vi "Update Low Limit.vi"(7 "BLRL Type":T1, 8 "error in (no error)":errorcluster, 9 "Low Limit":string, 10 "Channel":string, 11 "BluelinesRedlines in":refnum<class "BluelinesRedlines.lvclass">) -> (0 "error out":errorcluster, 3 "BluelinesRedlines out":refnum<class "BluelinesRedlines.lvclass">)   [LabVIEW 2020, in "VolatusGUIElements.lvlib" / "BluelinesRedlines.lvclass"]
uses:
  BluelinesRedlines.lvclass
  BluelinesRedlines.lvclass/BluelinesRedlines.ctl
  User BluelinesRedlines/User BluelinesRedlines.lvclass
  C:/dev/lv20CE/relink/lv-volatus/VolatusGUI/BluelinesRedlines Source/BluelinesRedlines Source.lvclass
  VolatusGUI/BluelinesRedlines Source/BLRL Type.ctl
  VolatusGUI/BluelinesRedlines Source/BluelinesRedlines Source.lvclass
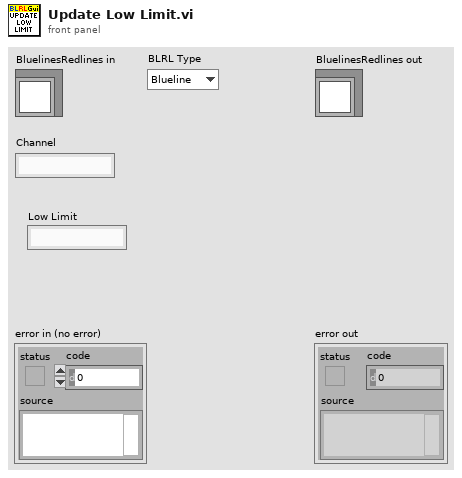
[diagram p1: front panel]
types:
  T1 = typedef "VolatusGUI.lvlib/BluelinesRedlines Source.lvclass/BLRL Type.ctl" = enum16{"Blueline", "Redline"}
  T2 = map{string, refnum<class "BluelinesRedlines Source.lvclass">}
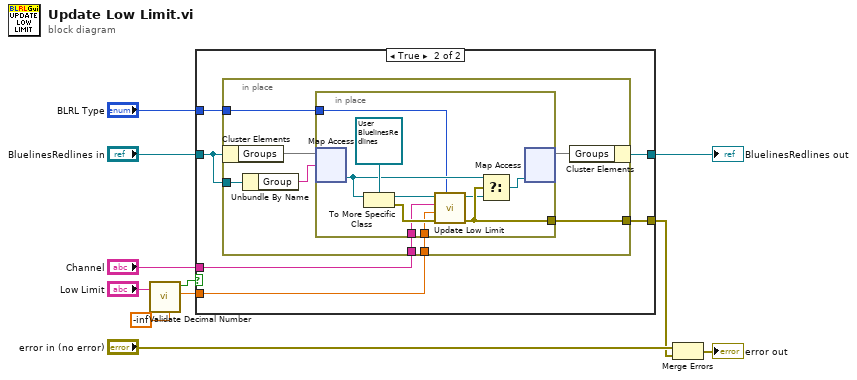
[diagram p0: block diagram]
diagram:
  n1 = call "Validate Decimal Number.vi"("String"="Low Limit", "Empty Default"=-inf) -> ("Valid"=w1:bool, "Value"=w3:dbl)  [unwired: 4 in]
  n2 = case shown="True" w1 {
    tunnel: "BluelinesRedlines in" -> [w12 w18]
    tunnel: [w12 w17] -> w9
    tunnel: "BLRL Type" -> [_ w16]
    tunnel: "Channel" -> [_ w15]
    tunnel: [_ w14] -> w4
    tunnel: w3 -> [_ w13]
    frame False {
    }
    frame True {
      n3 = in-place {
        in-place-border: w18 -> [w26]
        in-place-border: w15 -> [w22]
        in-place-border: w16 -> [w21]
        in-place-border: [w20] -> w14
        in-place-border: w13 -> [w19]
        n4 = in-place-cluster #1(w18) -> ("Groups"=w25:T2)
        n5 = Unbundle By Name(w26) -> ("Group"=w24:string)
        n6 = in-place {
          in-place-border: w22 -> [w30]
          in-place-border: w21 -> [w29]
          in-place-border: [w36] -> w20
          in-place-border: w19 -> [w27]
          n7 = in-place-map #2(w25, w24) -> (w33:refnum<class "BluelinesRedlines Source.lvclass">)  [unwired: 1 in, 1 out]
          n8 = To More Specific Class(target class=refnum<class "User BluelinesRedlines.lvclass"> refnum ("VolatusGUIElements.lvlib:User BluelinesRedlines.lvclass"), reference=w33) -> (specific class reference=w31:refnum<class "User BluelinesRedlines.lvclass">, error out=w35:errorcluster)  [unwired: 1 in]
          n9 = call "Update Low Limit.vi"("Type"=w29, "error in (no error)"=w35, "Low Limit"=w27, "Channel Name"=w30, "User BluelinesRedlines in"=w31) -> ("error out"=w36:errorcluster, "User BluelinesRedlines out"=w28:refnum<class "User BluelinesRedlines.lvclass">)  [unwired: 5 in]
          n10 = Select(t=w33, s=w36, f=w28) -> (s? t:f=w32:refnum<class "BluelinesRedlines Source.lvclass">)
          n11 = in-place-map #2(w32) -> (w23:T2)  [unwired: 1 in, 2 out]
        }
        n12 = in-place-cluster #1("Groups"=w23) -> (w17:refnum<class "BluelinesRedlines.lvclass">)
      }
    }
  }
  "BluelinesRedlines out" <- w9
  n13 = Merge Errors("error in (no error)", w4) -> (→"error out":errorcluster)
